vi "Run_Login.vi"(7 "Task":enum16{"Run", "Open"}(ring), 11 "Device":string) -> (0 "error out":errorcluster)   [LabVIEW 2016]
panel:
  out "appended path":path
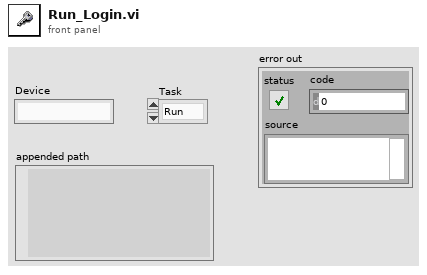
[diagram p1: front panel]
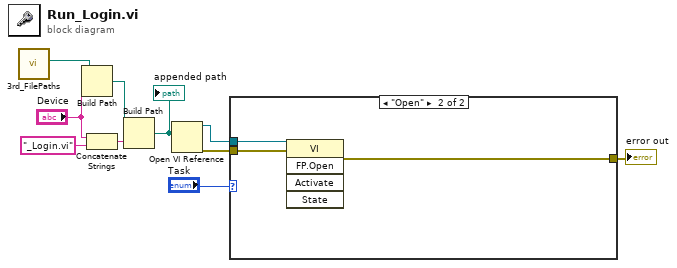
[diagram p0: block diagram]
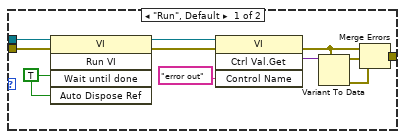
[diagram p2: hidden frame]
diagram:
  n1 = call "3rd_FilePaths.vi"() -> ("Device Folder"=w6:path)  [unwired: 9 in, 2 out]
  n2 = Build Path(base path=w6, name or relative path="Device") -> (appended path=w4:path)
  n3 = Concatenate Strings("Device", "_Login.vi" ("string")) -> (w7:string)
  n4 = Build Path(base path=w4, name or relative path=w7) -> (appended path=w9:path)
  "appended path" <- w9
  n5 = Open VI Reference(vi path=w9) -> (vi reference=w3:refnum<vi>, error out=w10:errorcluster)  [unwired: 5 in]
  n6 = case shown="\"Open\"" "Task" {
    tunnel: w10 -> [w21 w23]
    tunnel: w3 -> [w20 w24]
    tunnel: [w11 w22] -> w2
    frame "Run", Default {
      w19 = TRUE ("Wait Until Done")
      n7 = invoke class="VI" method="Run VI"(reference=w20, error in=w21, "Wait until done"=w19, "Auto Dispose Ref"=w19) -> (reference out=w18:refnum<vi>, error out=w16:errorcluster)  [unwired: 1 in, 3 out]
      n8 = invoke class="VI" method="Ctrl Val.Get"(reference=w18, error in=w16, "Control Name"="error out") -> (error out=w14:errorcluster, "Get Control Value Variant"=w15:variant)  [unwired: 1 in, 2 out]
      n9 = Variant To Data(type=w14, Variant=w15) -> (data=w13:errorcluster, error out=w12:errorcluster)  [unwired: 1 in]
      n10 = Merge Errors(w14, w13, w12) -> (w11:errorcluster)
    }
    frame "Open" {
      n11 = invoke class="VI" method="FP.Open"(reference=w24, error in=w23) -> (error out=w22:errorcluster)  [unwired: 3 in, 4 out]
    }
  }
  "error out" <- w2
